vi "DAQ.Write.vi"(8 "error in (no error)":errorcluster, 10 "Write":T1, 11 "DAQmx.AO in":refnum<class "DAQmx.AO.lvclass">) -> (0 "error out":errorcluster, 3 "DAQmx.AO out":refnum<class "DAQmx.AO.lvclass">)   [LabVIEW 2016, in "DAQmx.AO.lvclass"]
uses:
  DAQmx.AO.lvclass
  C:/user/patrick/hg/lockin.SMO/lvsrc/DAQmx/DAQmx.lvclass
  DAQ/Typedefs/PrivateEvents--DAQ.Write.ctl
  DAQmx/DAQmx.lvclass/DAQmx.ctl
  <vilib>/DAQmx/write.llb/DAQmx Write (Analog 1D Wfm NChan NSamp).vi
  <vilib>/DAQmx/miscellaneous.llb/DAQmx Fill In Error Info.vi
  <resource>/objmgr/daqmx.rc
  DAQmx/DAQmx.lvclass
  DAQ/DAQ.lvclass
panel:
  out "number of samples written per channel":u32
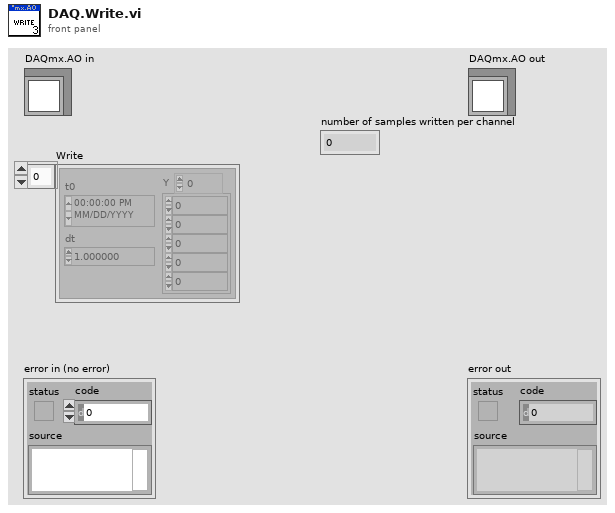
[diagram p1: front panel]
types:
  T1 = typedef "DAQ.lvclass/PrivateEvents--DAQ.Write.ctl" = waveform(dbl)[]
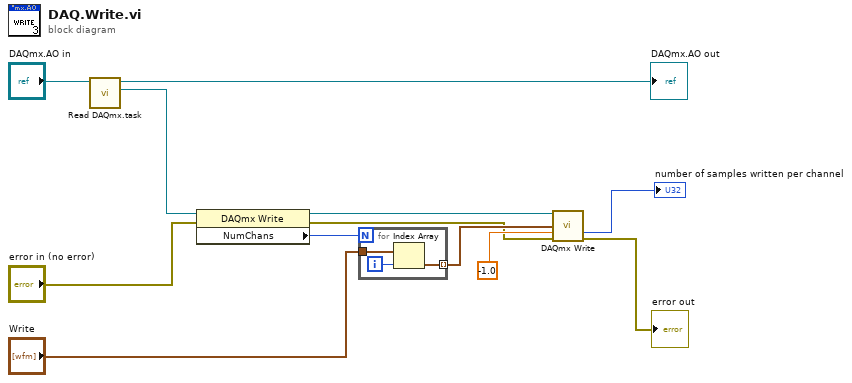
[diagram p0: block diagram]
diagram:
  n1 = call "Read DAQmx.task.vi"("DAQmx in"="DAQmx.AO in") -> ("task"=w6:refnum<k21>, "DAQmx out"=→"DAQmx.AO out":refnum<class "DAQmx.AO.lvclass">)  [unwired: 8 in, 1 out]
  n2 = property class="DAQmx Write"(reference=w6, error in="error in (no error)") -> (reference out=w11:refnum<k21>, error out=w3:errorcluster, "NumChans"=w12:u32)
  n3 = for {
    N: w12 -> [_]
    tunnel: "Write" -> [w15]
    tunnel: [w14] -> w10 mode=indexing
    i -> [w13]
    n4 = Index Array(array=w15, index=w13) -> (element=w14:waveform(dbl))
  }
  n5 = call-poly <vilib>:"DAQmx Write.vi"("task/channels in"=w11, "data"=w10, "timeout"=-1.0, "error in"=w3) -> ("number of samples written per channel"=→"number of samples written per channel":u32, "error out"=→"error out":errorcluster)  [unwired: 9 in, 1 out]
